vi "Hello_World.vi"   [LabVIEW 2018]
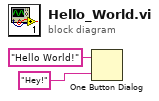
[diagram p0: block diagram]
diagram:
  n1 = One Button Dialog(message="Hello World!", button name ("OK")="Hey!") -> ()  [unwired: 1 out]
